vi "Find Workspace.vi"(8 "Error In":errorcluster, 10 "Control In":T2={"I-O.lvclass"=refnum, "Motion.lvclass"=refnum, "Dispenser.lvclass"=refnum}, 11 "Baseplate Tray in":refnum<class "Baseplate Tray.lvclass">) -> (0 "Error Out":errorcluster, 1 "Workspace":T1, 2 "Control Out":T2, 3 "Baseplate Tray Out":refnum<class "Baseplate Tray.lvclass">)   [LabVIEW 2016, in "Baseplate Tray.lvclass"]
uses:
  Baseplate Tray.lvclass
  C:/Users/HEP Gantry/Documents/GitHub/UCSB-Gantry/V5/Classes/Workspace/Fixture.lvclass
  Controller/Controllers.ctl
  Controller/I-O/I-O.lvclass
  Controller/Motion/A3200/A3200.lvclass
  Controller/Dispenser/Dispenser.lvclass
  Controller/Motion/Motion.lvclass
  Workspace.ctl
  Fixture.lvclass/Fixture.ctl
  Baseplate Tray.lvclass/Baseplate Tray.ctl
  Read Fixture ID.vi
  Fixture.lvclass
  Controller/Controller.lvclass
panel:
  in  "output cluster 2":T1
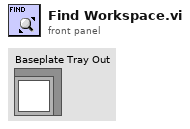
[diagram p1: front panel]
types:
  T1 = typedef "Fixture.lvclass/Workspace.ctl" = cluster{"XYZTheta":dbl[], "Workspace Valve":i32, "Workspace Sensor":i32}
  T2 = typedef "Controller.lvclass/Controllers.ctl" = cluster{"I-O.lvclass":refnum<class "I-O.lvclass">, "Motion.lvclass":refnum<class "Motion.lvclass">, "Dispenser.lvclass":refnum<class "Dispenser.lvclass">}
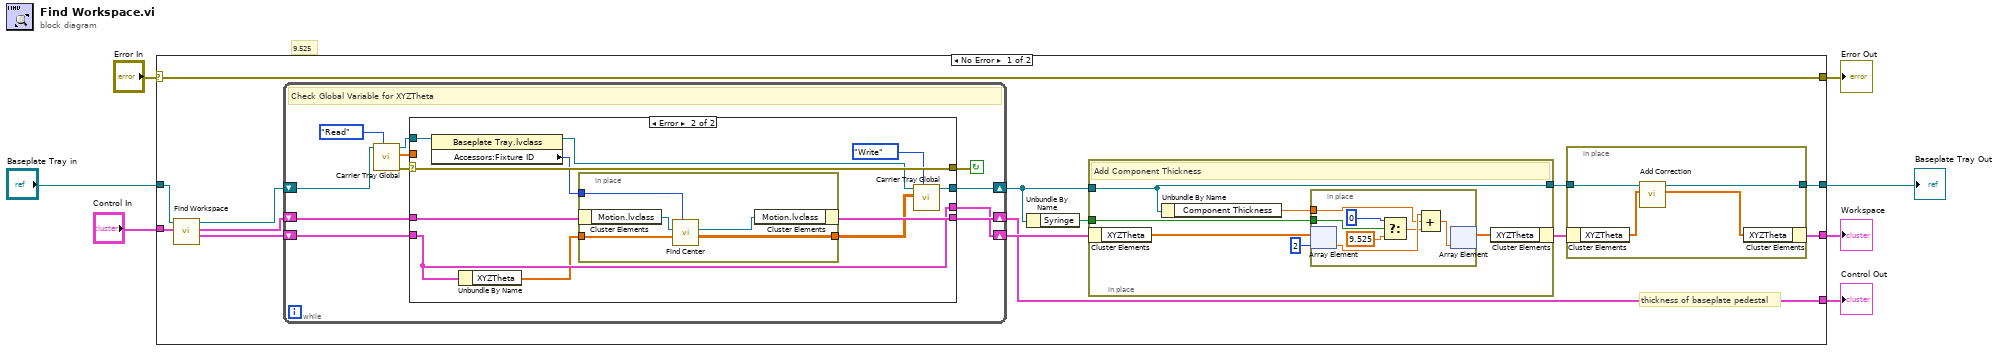
[diagram p0: block diagram]
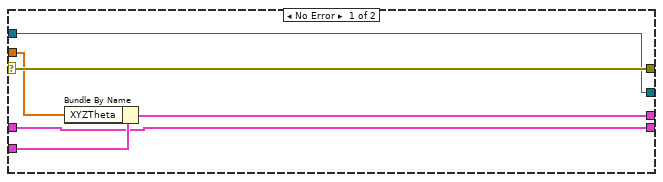
[diagram p2: hidden frame]
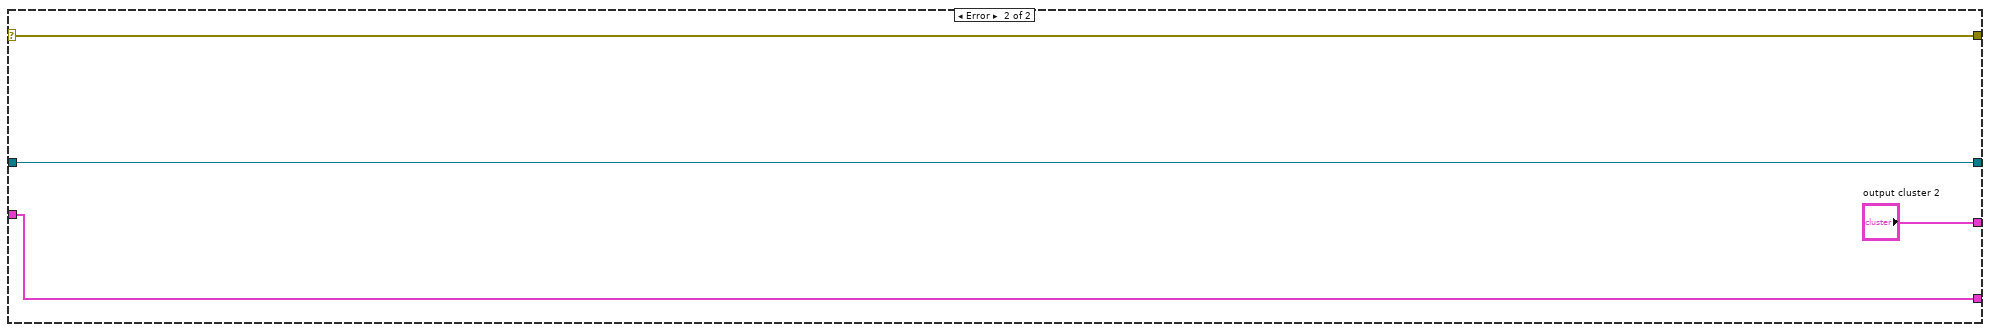
[diagram p3: hidden frame]
diagram:
  # "9.525"
  n1 = case shown="No Error" "Error In" {
    selector: "Error In" -> [w21 w74]
    tunnel: [w21 w74] -> w6
    tunnel: "Control In" -> [w20 w75]
    tunnel: [w14 w75] -> w4
    tunnel: "Baseplate Tray in" -> [w19 w72]
    tunnel: [w17 "output cluster 2"] -> w2
    tunnel: [w18 w72] -> w1
    frame No Error {
      # "thickness of baseplate pedestal"
      n2 = call-parent "Find Workspace.vi"("Control In"=w20, "Workspace In"=w19) -> (1:"Workspace Out"=w11:T1, "Control Out"=w10:T2, 3:"Workspace Out"=w12:refnum<class "Baseplate Tray.lvclass">)  [unwired: 6 in, 1 out]
      n3 = while {
        shift-right: [w27] -> w9
        shift-left: w12 -> [w35]
        shift-right: [w29] -> w14
        shift-left: w10 -> [w30]
        shift-right: [w26] -> w15
        shift-left: w11 -> [w31]
        stop <- w33 continue-if-true
        # "Check Global Variable for XYZTheta"
        n4 = call "Carrier Tray Global.vi"("Action"=enum16{"Initialize", "Read", "Write"}."Read", "Carrier Tray.lvclass"=w35) -> ("error out"=w34:errorcluster, "XYZTheta out"=w32:dbl[], "Carrier Tray.lvclass 2"=w28:refnum<class "Baseplate Tray.lvclass">)  [unwired: 7 in]
        n5 = case shown="Error" w34 {
          selector: w34 -> [w42 w53]
          tunnel: [w42 w53] -> w33
          tunnel: w32 -> [w41 _]
          tunnel: [w40 w47] -> w26
          tunnel: w31 -> [w39 w47]
          tunnel: w30 -> [w37 w52]
          tunnel: [w37 w51] -> w29
          tunnel: w28 -> [w38 w45]
          tunnel: [w38 w50] -> w27
          frame No Error {
            n6 = Bundle By Name(cluster=w39, "XYZTheta"=w41) -> (w40:T1)
          }
          frame Error {
            n7 = property class="Baseplate Tray.lvclass"(reference=w45) -> (reference out=w44:refnum<class "Baseplate Tray.lvclass">, "Accessors:Fixture ID"=w43:i32)  [unwired: 1 in, 1 out]
            n8 = Unbundle By Name(w47) -> ("XYZTheta"=w46:dbl[])
            n9 = in-place {
              in-place-border: [w56] -> w48
              in-place-border: w46 -> [w55]
              in-place-border: w43 -> [w54]
              n10 = in-place-cluster #1(w52) -> ("Motion.lvclass"=w57:refnum<class "Motion.lvclass">)
              n11 = call "Find Center.vi"("Tray Number"=w54, "XYZTheta"=w55, "Motion.lvclass"=w57) -> ("XYZTheta Centers"=w56:dbl[][], "Motion Out"=w58:refnum<class "Motion.lvclass">)  [unwired: 7 in]
              n12 = in-place-cluster #1("Motion.lvclass"=w58) -> (w51:T2)
            }
            n13 = call "Carrier Tray Global.vi"("Action"=enum16{"Initialize", "Read", "Write"}."Write", "XYZTheta in"=w48, "Carrier Tray.lvclass"=w44) -> ("Carrier Tray.lvclass 2"=w50:refnum<class "Baseplate Tray.lvclass">)  [unwired: 6 in, 2 out]
          }
        }
      }
      n14 = Unbundle By Name(w9) -> ("Syringe"=w8:bool)
      n15 = in-place {
        in-place-border: w9 -> [w60]
        in-place-border: [w60] -> w13
        in-place-border: w8 -> [w59]
        # "Add Component Thickness"
        n16 = in-place-cluster #2(w15) -> ("XYZTheta"=w63:dbl[])
        n17 = Unbundle By Name(w60) -> ("Component Thickness"=w61:dbl)
        n18 = in-place {
          in-place-border: w61 -> [w70]
          in-place-border: w59 -> [w68]
          n19 = in-place-array #3(w63, 2) -> (w71:dbl)
          n20 = Select(t=0, s=w68, f=9.525) -> (s? t:f=w65:dbl)
          n21 = Compound Arithmetic op=ADD(w71, w70, w65) -> (w69:dbl)
          n22 = in-place-array #3(w69) -> (w62:dbl[])  [unwired: 1 out]
        }
        n23 = in-place-cluster #2("XYZTheta"=w62) -> (w16:T1)
      }
      n24 = in-place {
        in-place-border: [w25] -> w18
        in-place-border: w13 -> [w24]
        n25 = in-place-cluster #4(w16) -> ("XYZTheta"=w23:dbl[])
        n26 = call "Add Correction.vi"("XYZTheta"=w23, "Carrier Tray in"=w24) -> ("XYZTheta Out"=w22:dbl[], "Carrier Tray out"=w25:refnum<class "Baseplate Tray.lvclass">)  [unwired: 7 in, 1 out]
        n27 = in-place-cluster #4("XYZTheta"=w22) -> (w17:T1)
      }
    }
    frame Error {
    }
  }
  "Error Out" <- w6
  "Control Out" <- w4
  "Workspace" <- w2
  "Baseplate Tray Out" <- w1
